vi "Extract Green Plane.vi"(8 "error in (no error)":errorcluster, 10 "target":T1, 11 "source":T1) -> (0 "error out":errorcluster, 3 "target":T1)   [LabVIEW 2014]
doc: "Extracts the sclera plane and puts it into the specified buffer image."
uses:
  <vilib>/vision/Image Controls.llb/IMAQ Image.ctl
  <vilib>/vision/NI_Vision_Development_Module.lvlib
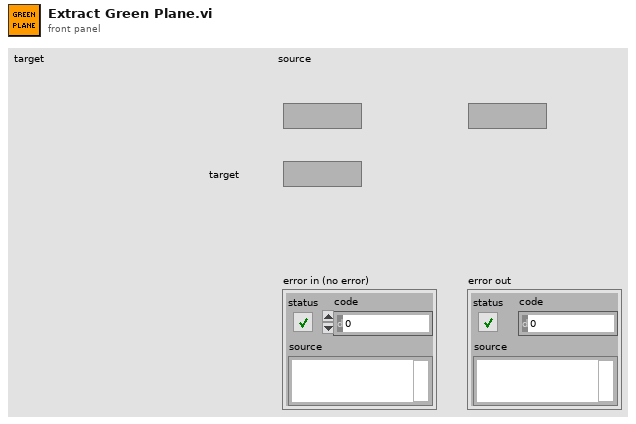
[diagram p1: front panel]
types:
  T1 = typedef "IMAQ Image.ctl" = refnum<image>
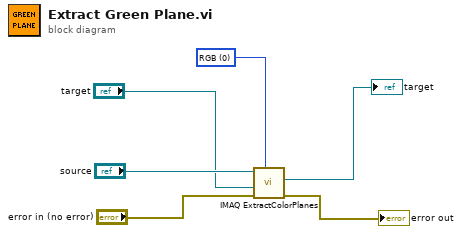
[diagram p0: block diagram]
diagram:
  w1 = u16 0 items=["RGB", "HSL", "HSV", "HSI"] ("Color Mode")
  n1 = call "IMAQ ExtractColorPlanes"("Color Mode"=w1, "error in (no error)"="error in (no error)", "Green or Sat Plane"="target", "Image Src"="source") -> ("error out"=→"error out":errorcluster, "Green or Sat Plane out"=→"target":T1)  [unwired: 4 in, 2 out]
